vi "QLCDemoCustom.vi"() -> ()   [LabVIEW 2017]
uses:
  <userlib>/QLC/QLC.lvlib
panel:
  in  "Gaze Vector Number":dbl=1.0
  out "Gaze Vector\nOverflow":bool
  out "Gaze Vector":sgl[](graph)
  out "Gaze Vector Number":dbl
  out "Camera Time":i32
  out "Hour":i32
  out "Sec/10":i32
  out "Min":i32
  out "Year":i32
  out "Day":i32
  out "Sec":i32
  out "Camera Time":bool
  out "IRIG":bool
  out "SMPTE":bool
  out "Analog Data Overflow":bool
  out "Camera Timestamp":u64
  out "Camera Frame Number":u32
  out "Analog samples":dbl
  out "Analog frame nr":dbl
  out "Analog":sgl[](graph)
  in  "Save Filename":string
  in  "Save Capture":bool caption="Stop Capture"
  in  "Event Label":string
  in  "Send Trig":bool
  in  "Set Event":bool
  in  "Stop Capture":bool
  in  "Close Measurement":bool
  in  "New Measurement":bool caption="Start Measurement"
  in  "Control QTM":bool caption="Off   On"
  out "Controlling QTM":bool
  in  "Start RT From File":bool
  in  "Start Capture":bool
  out "Analog value":dbl
  in  "Analog Channel":dbl=1.0
  in  "Analog Device":dbl=1.0
  out "AnalogSingle":sgl(graph)
  in  "6 DOF Body":i32(knob)=1 min=1 max=5 step=1 scale=1.0..5.0
  out "Pitch":sgl(graph)
  out "Roll":sgl(graph)
  out "3D Z":dbl(knob) scale=0.0..300.0
  out "3D Y":dbl(knob) scale=-1200.0..1200.0
  out "3D X":dbl(knob) scale=0.0..1200.0
  in  "Connect to QTM":bool
  out "Last QTM Event":dbl=2.0
  out "Yaw":sgl(graph)
  out "3D Z":dbl
  out "3D Y":dbl
  out "3D X":dbl
  in  "3D Marker":i32(knob)=1 min=1 max=13 step=1 scale=1.0..13.0
  out "QTM Message":string="QTM connection closed"
  in  "Data":string="3D 6DEuler Analog AnalogSingle GazeVector Timecode"
  in  "Frequency":string="AllFrames"
  in  "Port":i32=22222 min=22222 max=65535
  in  "Address":string="192.168.16.100"
  # "Usage: [FrequencyDivisor:n] [Frequency:n] [AllFrames]    (No value equals polling mode)"
  # "Usage: [All] [2D] [3D] [3DRes] [3DnoLabels] [3DnoLabelsRes] [Analog] [AnalogSingle]\n             [Force] [ForceSingle] [6D] [6DRes] [6DEuler] [6DEulerRes] [GazeVector] [Timecode]"
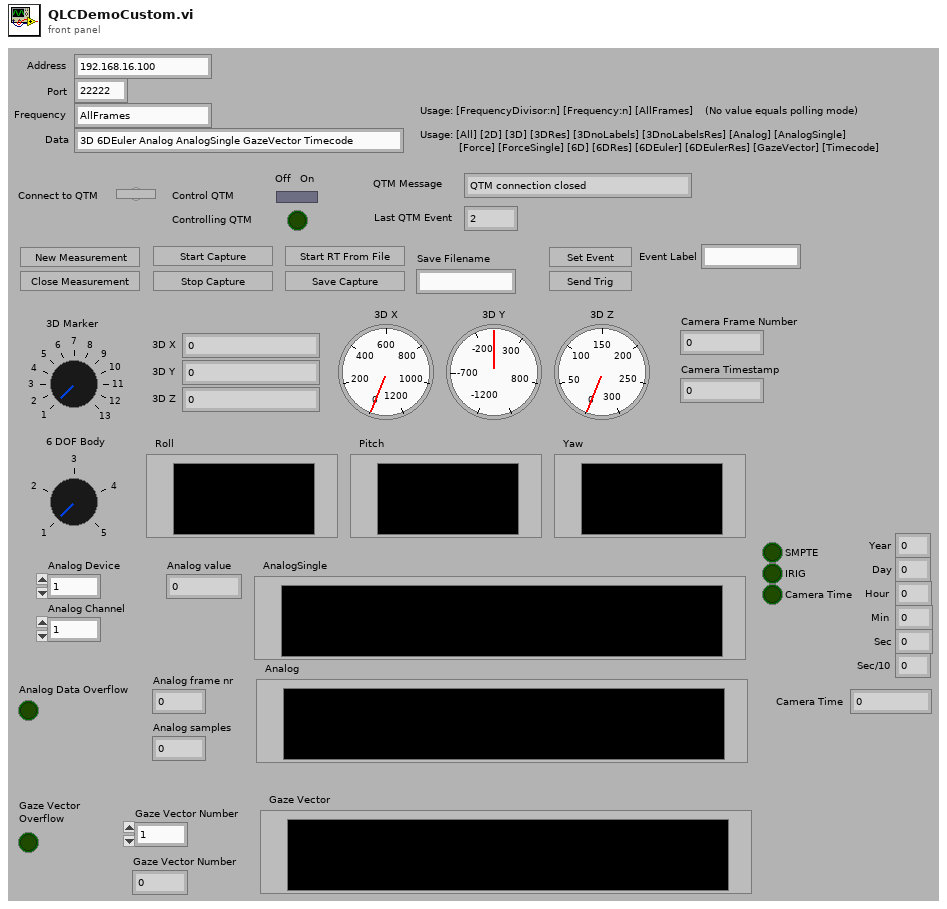
[diagram p1: front panel]
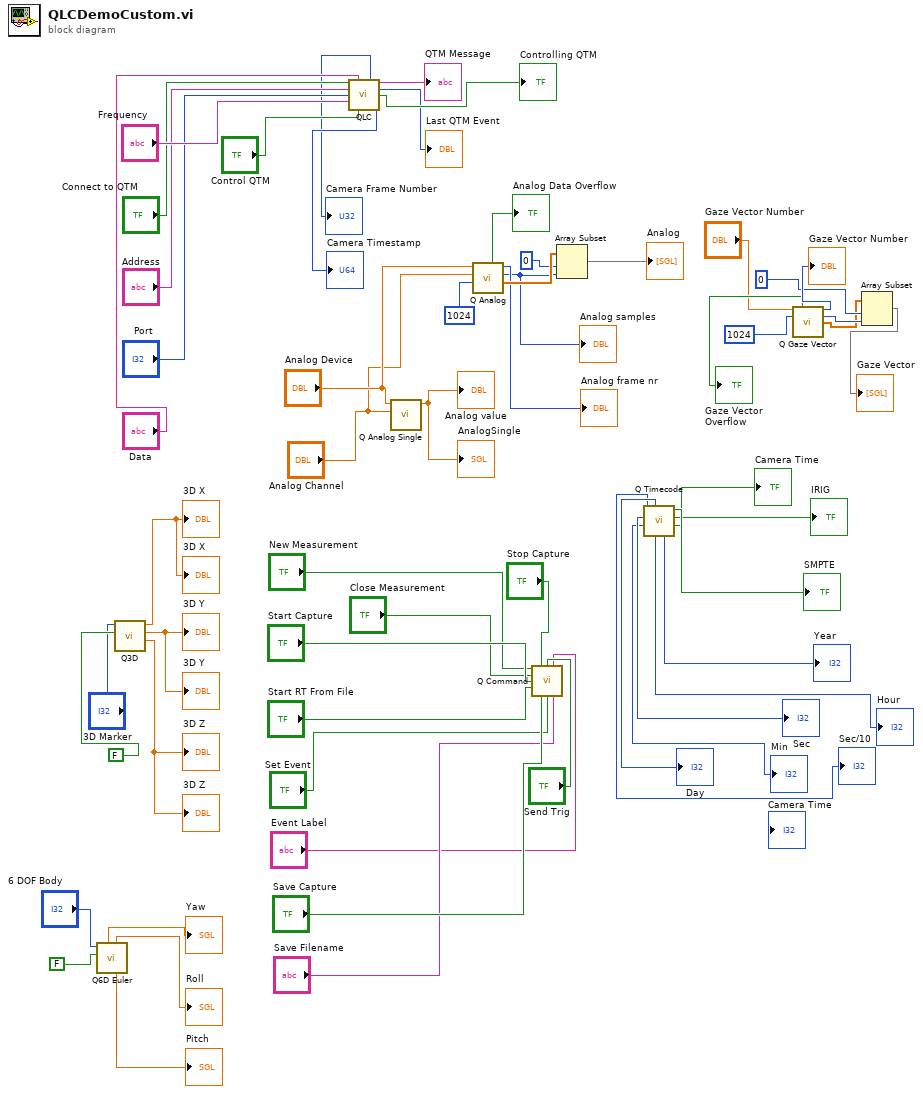
[diagram p0: block diagram]
diagram:
  n1 = call <userlib>:"Q6D Euler.vi"("residual"=FALSE, "no"="6 DOF Body") -> ("pitch"=→"Pitch":sgl, "roll"=→"Roll":sgl, "yaw"=→"Yaw":sgl)  [unwired: 3 in, 4 out]
  n2 = call <userlib>:"Q3D.vi"("residual"=FALSE, "no"="3D Marker") -> ("z"=→"3D Z" →"3D Z":sgl, "y"=→"3D Y" →"3D Y":sgl, "x"=→"3D X" →"3D X":sgl)  [unwired: 6 in, 1 out]
  n3 = call <userlib>:"QLC.vi"("connect"="Connect to QTM", "data"="Data", "address"="Address", "port"="Port", "frequency"="Frequency", "controlQTM"="Control QTM") -> ("camFrameNumber"=→"Camera Frame Number":u32, "message"=→"QTM Message":string, "lastEvent"=→"Last QTM Event":i32, "QTMMaster"=→"Controlling QTM":bool, "camTimeStamp"=→"Camera Timestamp":u64)  [unwired: 4 in, 1 out]
  n4 = call <userlib>:"Q Analog Single.vi"("channel"="Analog Channel", "device"="Analog Device") -> ("v"=→"AnalogSingle" →"Analog value":sgl)  [unwired: 9 in]
  n5 = call <userlib>:"Q Analog.vi"("dataSize"=1024, "channel"="Analog Channel", "device"="Analog Device") -> ("data"=w43:sgl[], "sampleCount"=w39:i32, "sampleNumber"=→"Analog frame nr":i32, "overflow"=→"Analog Data Overflow":bool)  [unwired: 5 in]
  "Analog samples" <- w39
  n6 = call <userlib>:"Q Command.vi"("bNew"="New Measurement", "bStop"="Stop Capture", "bTrig"="Send Trig", "pEventLabel"="Event Label", "bClose"="Close Measurement", "bStart"="Start Capture", "bStartFile"="Start RT From File", "bSave"="Save Capture", "bEvent"="Set Event", "pFileName"="Save Filename") -> ()  [unwired: 5 in, 1 out]
  n7 = Array Subset(array=w43, index=0, length=w39) -> (→"Analog":sgl[])
  n8 = call <userlib>:"Q Timecode.vi"() -> ("camTime"=→"Camera Time":bool, "irig"=→"IRIG":bool, "smpte"=→"SMPTE":bool, "year"=→"Year":i32, "hour"=→"Hour":i32, "day"=→"Day":i32, "minute"=→"Min":i32, "second"=→"Sec":i32, "frameTenth"=→"Sec/10":i32)  [unwired: 2 in, 1 out]
  n9 = call <userlib>:"Q Gaze Vector.vi"("no"="Gaze Vector Number", "dataSize"=1024) -> ("overflow"=→"Gaze Vector\nOverflow":bool, "gazeVectorNumber"=→"Gaze Vector Number":i32, "gazeVectorCount"=w7:i32, "x"=w6:sgl[])  [unwired: 5 in, 5 out]
  n10 = Array Subset(array=w6, index=0, length=w7) -> (→"Gaze Vector":sgl[])
